vi "Camera.vi"(7 "Machine Vision":T1=enum."Tray Fiducials", 8 "error in (no error)":errorcluster, 10 "Stop":bool, 11 "Camera in":refnum<class "Camera.lvclass">) -> (0 "error out":errorcluster, 1 "Camera":dbl[](array[numeric]), 2 "Image":T2(plugin-control), 3 "Camera out":refnum<class "Camera.lvclass">)   [LabVIEW 2016, in "Camera.lvclass"]
uses:
  Camera.lvclass
  Machine Vision.ctl
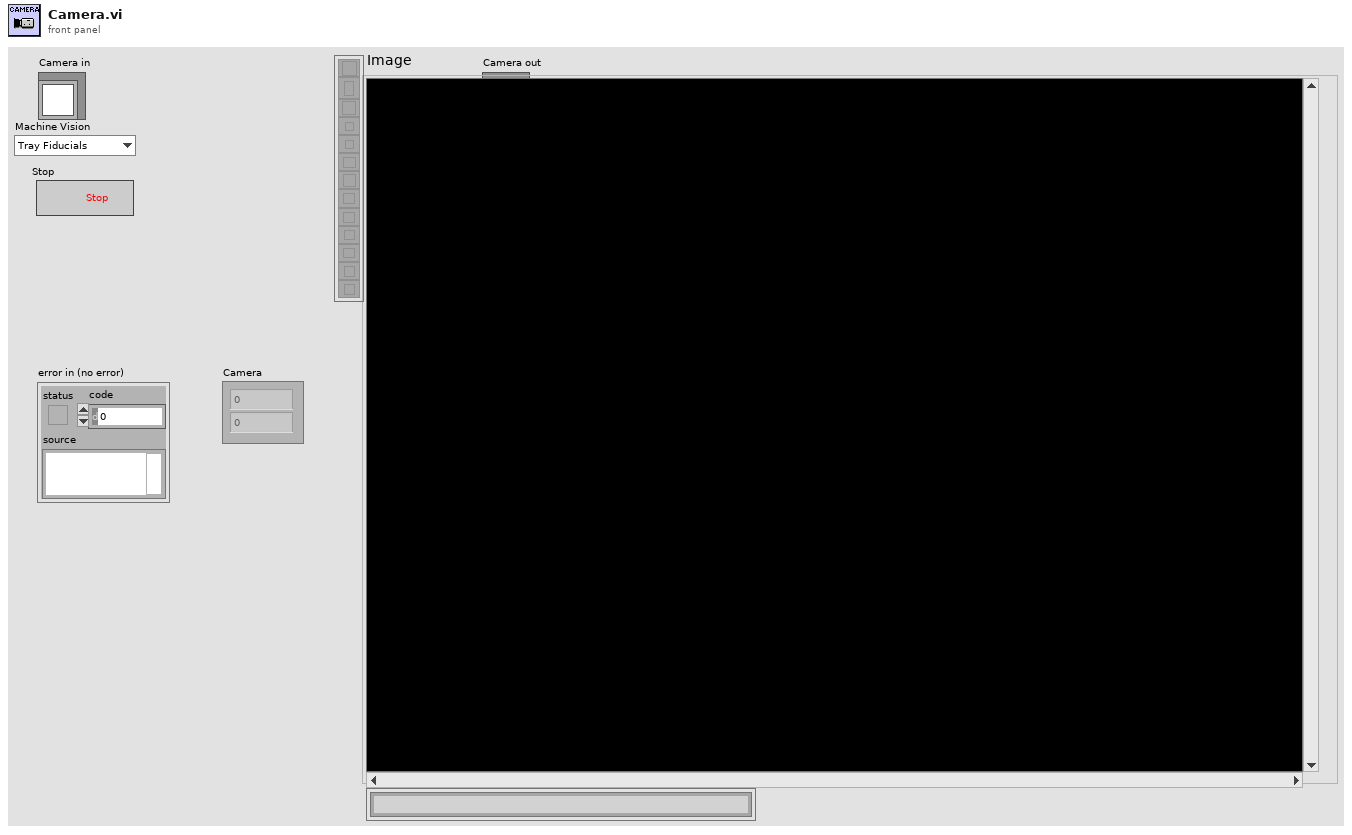
[diagram p1: front panel]
types:
  T1 = typedef "Camera.lvclass/Machine Vision.ctl" = enum16{"None", "Tray Fiducials", "HPK Silicon", "Hexaboard", "Corner (TL, BR)", "Corner (BL, TR)"}
  T2 = typedef "IMAQ Image.ctl" = refnum<image>
  T3 = cluster{"Center (Pixels)":cluster{"X":sgl, "Y":sgl}, "Radius (Pixels)":dbl, "Center (Real-World)":cluster{"X":sgl, "Y":sgl}, "Radius (Real-World)":dbl, "Roundness (Real-World)":dbl, "Average Strength":dbl, "Average SNR (dB)":dbl}
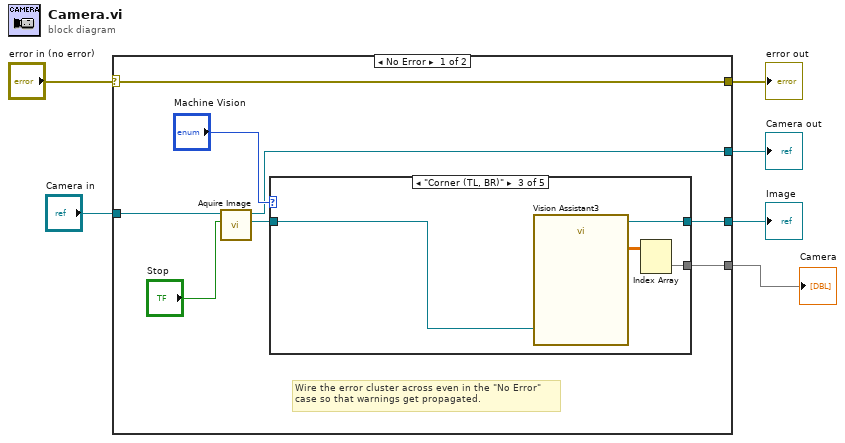
[diagram p0: block diagram]
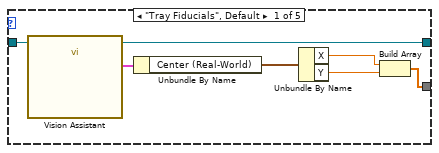
[diagram p2: hidden frame]
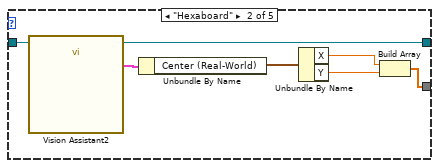
[diagram p3: hidden frame]
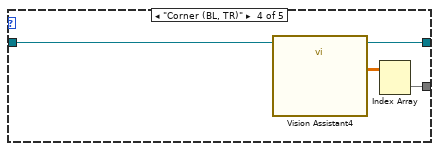
[diagram p4: hidden frame]
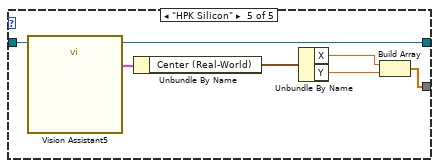
[diagram p5: hidden frame]
diagram:
  n1 = case shown="No Error" "error in (no error)" {
    selector: "error in (no error)" -> [w14 w45]
    tunnel: [w14 w45] -> w5
    tunnel: [w10 w44] -> w4
    tunnel: "Camera in" -> [w11 w44]
    tunnel: [w9 _] -> w2
    tunnel: [w8 _] -> w1
    frame No Error {
      # "Wire the error cluster across even in the \"No Error\"\ncase so that warnings get propagated."
      n2 = call-dynamic "Aquire Image.vi"("Stop"="Stop", "Camera in"=w11) -> ("Image Out"=w7:T2, "Camera out"=w10:refnum<class "Camera.lvclass">)  [unwired: 7 in, 1 out]
      n3 = case shown="\"Corner (TL, BR)\"" "Machine Vision" {
        tunnel: [w17 w22 w29 w33 w38] -> w9
        tunnel: [w20 w23 w32 w36 w40] -> w8
        tunnel: w7 -> [w21 w24 w31 w35 w39]
        frame "Tray Fiducials", Default {
          n4 = call "Vision Assistant"("Image In"=w21) -> ("Image Out"=w20:T2, "Fitted Circle (Find Circular Edge 1)"=w16:T3)  [unwired: 24 in, 1 out]
          n5 = Unbundle By Name(w16) -> ("Center (Real-World)"=w19:cluster{"X":sgl, "Y":sgl})
          n6 = Unbundle By Name(w19) -> ("X"=w18:sgl, "Y"=w15:sgl)
          n7 = Build Array(w18, w15) -> (w17:sgl[])
        }
        frame "Hexaboard" {
          n8 = call "Vision Assistant2"("Image In"=w24) -> ("Image Out"=w23:T2, "Fitted Circle (Find Circular Edge 1)"=w26:T3)  [unwired: 24 in, 1 out]
          n9 = Unbundle By Name(w26) -> ("Center (Real-World)"=w28:cluster{"X":sgl, "Y":sgl})
          n10 = Unbundle By Name(w28) -> ("X"=w27:sgl, "Y"=w25:sgl)
          n11 = Build Array(w27, w25) -> (w22:sgl[])
        }
        frame "Corner (TL, BR)" {
          n12 = call "Vision Assistant3"("Image In"=w31) -> ("Image Out"=w32:T2, "Calibrated Results (Top Left, Bottom Right)"=w30:sgl[][])  [unwired: 23 in, 2 out]
          n13 = Index Array(array=w30) -> (element=w29:sgl[])  [unwired: 2 in]
        }
        frame "Corner (BL, TR)" {
          n14 = call "Vision Assistant4"("Image In"=w35) -> ("Image Out"=w36:T2, "Calibrated Results (Bottom Left, Top Right)"=w34:sgl[][])  [unwired: 23 in, 2 out]
          n15 = Index Array(array=w34) -> (element=w33:sgl[])  [unwired: 2 in]
        }
        frame "HPK Silicon" {
          n16 = call "Vision Assistant5"("Image In"=w39) -> ("Image Out"=w40:T2, "Fitted Circle (Find Circular Edge 1)"=w37:T3)  [unwired: 24 in, 1 out]
          n17 = Unbundle By Name(w37) -> ("Center (Real-World)"=w43:cluster{"X":sgl, "Y":sgl})
          n18 = Unbundle By Name(w43) -> ("X"=w42:sgl, "Y"=w41:sgl)
          n19 = Build Array(w42, w41) -> (w38:sgl[])
        }
      }
    }
    frame Error {
    }
  }
  "error out" <- w5
  "Camera out" <- w4
  "Camera" <- w2
  "Image" <- w1
